vi "CombinePNGsStackedArray.vi"(8 "error in (no error)":errorcluster, 10 "Output File":path, 11 "Input Files":path[](array[path])) -> (0 "error out":errorcluster)   [LabVIEW 2020, in "VIDiffScreenshots.lvlib"]
uses:
  VIDiffScreenshots.lvlib
  ImageMagic/Append Method.ctl
  ImageMagic/VIDiffImageMagic.lvlib
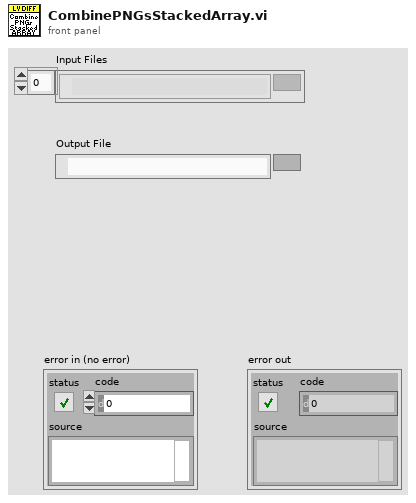
[diagram p1: front panel]
types:
  T1 = typedef "VIDiffImageMagic.lvlib/Append Method.ctl" = enum16{"Vertical", "Horizontal"}
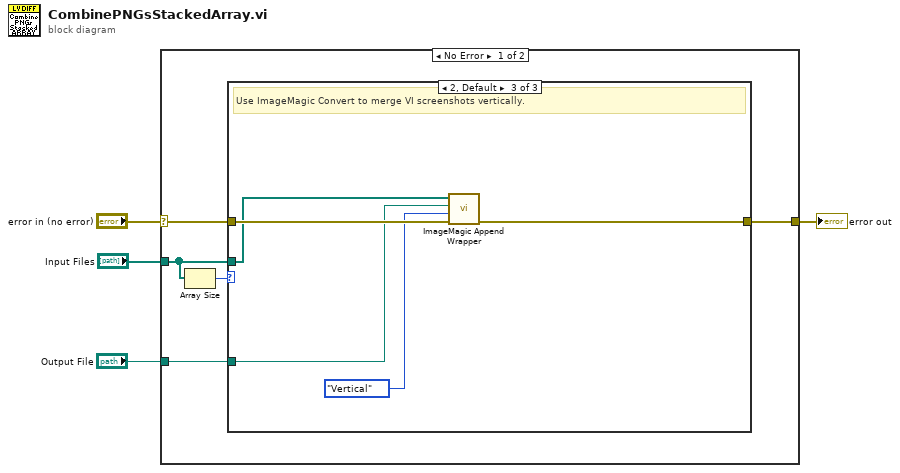
[diagram p0: block diagram]
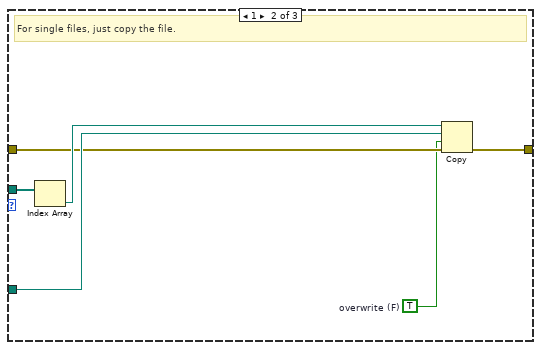
[diagram p3: hidden frame]
diagram:
  n1 = case shown="No Error" "error in (no error)" {
    selector: "error in (no error)" -> [w7 w22]
    tunnel: "Input Files" -> [w5 _]
    tunnel: [w9 w22] -> w2
    tunnel: "Output File" -> [w8 _]
    frame No Error {
      n2 = Array Size(array=w5) -> (size(s)=w6:i32)
      n3 = case shown="2, Default" w6 {
        tunnel: [w10 w11 w20] -> w9
        tunnel: w8 -> [_ w14 w18]
        tunnel: w7 -> [w10 w13 w21]
        tunnel: w5 -> [_ w16 w19]
        frame 0 {
          # "Do nothing."
        }
        frame 1 {
          w12 = TRUE  # overwrite (F)
          # "For single files, just copy the file."
          n4 = Index Array(array=w16) -> (element=w15:path)  [unwired: 1 in]
          n5 = Copy(8:w13, 9:w12, 10:w14, 11:w15) -> (0:w11:errorcluster)  [unwired: 1 in, 2 out]
        }
        frame 2, Default {
          # "Use ImageMagic Convert to merge VI screenshots vertically."
          n6 = call "ImageMagic Append Wrapper.vi"("error in (no error)"=w21, "Append Method"=Append_Method."Vertical", "Output File"=w18, "Input Files"=w19) -> ("error out"=w20:errorcluster)  [unwired: 7 in]
        }
      }
    }
    frame Error {
    }
  }
  "error out" <- w2
